vi "sweep -- generate freqs.vi"(9 "sweep parameters":T1={"scan type"=enum."linear", "N"=-1, "cursor window"={"left"=2378.60310421286, "right "=2421.6740576496672, "center"=2421.6740576496672, "window"=2421.6740576496672, "cursors"=[], "relative"=0, "absolute"=0, "fixed vertical offset"=2421.6740576496672, "vertical offset"=2421.6740576496672, "skew"=2421.6740576496672, "default window frac"=2421.6740576496672, "kind"=enum."skewed", "skew.left"=2421.6740576496672, "skew.right"=2421.6740576496672, "Plot ref"=refnum, "wing order"=enum."back"}}) -> (2 "Array":dbl[](array[numeric]))   [LabVIEW 2017]
uses:
  sweep parameters.ctl
  cursor winow.ctl
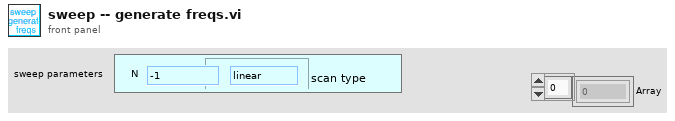
[diagram p1: front panel]
types:
  T1 = typedef "sweep parameters.ctl" = cluster{"scan type":enum16{"linear", "arctan"}, "N":i64, "cursor window":T2}
  T2 = typedef "cursor winow.ctl" = cluster{"left":dbl, "right ":dbl, "center":dbl, "window":dbl, "cursors":i32[], "relative":i32, "absolute":i32, "fixed vertical offset":dbl, "vertical offset":dbl, "skew":dbl, "default window frac":dbl, "kind":enum16{"symmetric", "skewed", "fancy"}, "skew.left":dbl, "skew.right":dbl, "Plot ref":refnum<vi>, "wing order":enum16{"forw", "back"}}
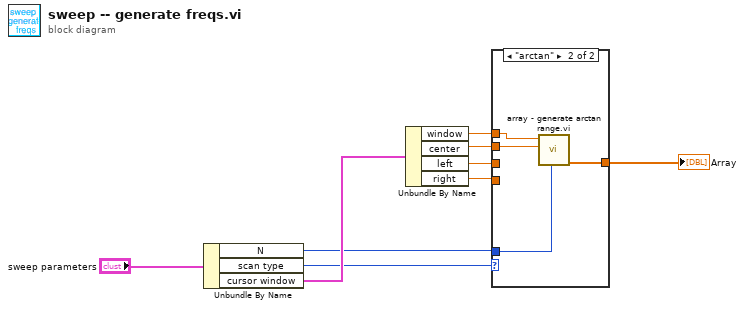
[diagram p0: block diagram]
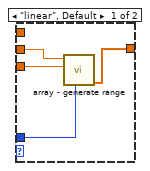
[diagram p2: hidden frame]
diagram:
  n1 = Unbundle By Name("sweep parameters") -> ("N"=w4:i64, "scan type"=w5:enum16{"linear", "arctan"}, "cursor window"=w6:T2)
  n2 = Unbundle By Name(w6) -> ("window"=w2:dbl, "center"=w1:dbl, "left"=w8:dbl, "right"=w7:dbl)
  n3 = case shown="\"arctan\"" w5 {
    tunnel: [w13 w17] -> w9
    tunnel: w8 -> [w12 _]
    tunnel: w7 -> [w11 _]
    tunnel: w4 -> [w10 w16]
    tunnel: w2 -> [_ w15]
    tunnel: w1 -> [_ w14]
    frame "linear", Default {
      n4 = call "array - generate range.vi"("N"=w10, "freq max"=w11, "freq min"=w12) -> ("Array"=w13:dbl[])  [unwired: 7 in, 1 out]
    }
    frame "arctan" {
      n5 = call "array - generate arctan range.vi.vi"("N"=w16, "omega0"=w14, "gamma"=w15) -> ("Array"=w17:dbl[])  [unwired: 8 in]
    }
  }
  "Array" <- w9
